vi "getFAs.vi"(11 "ILCCommunications in":refnum<class "ILCCommunications.lvclass">) -> (2 "FAs":refnum<class "FAILC.lvclass">[](array[class]), 3 "ILCCommunications out":refnum<class "ILCCommunications.lvclass">)   [LabVIEW 2016, in "ILCCommunications.lvclass"]
uses:
  ILCCommunications.lvclass
  Common_RT_FAILC/FAILC/FAILC.lvclass
  ILCCommunications.lvclass/ILCCommunications.ctl
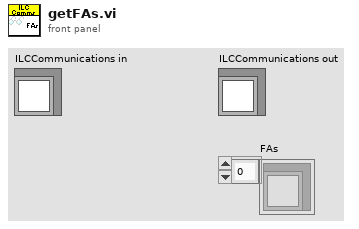
[diagram p1: front panel]
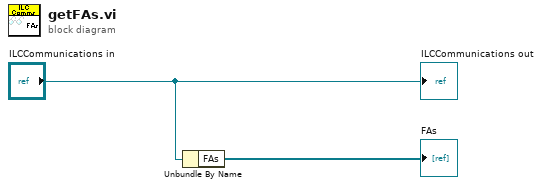
[diagram p0: block diagram]
diagram:
  n1 = Unbundle By Name("ILCCommunications in") -> ("FAs"=→"FAs":refnum<class "FAILC.lvclass">[])
  "ILCCommunications out" <- "ILCCommunications in"
